vi "SENS_SEGM_STAT_ON_OFF.vi"(0 "VISA IN":refnum<visa-resource-name>, 1 "Segment":i32, 2 "Segment ON/OFF":bool, 5 "error in":errorcluster, 7 "Channel":i32) -> (14 "VISA Out":refnum<visa-resource-name>, 19 "error out":errorcluster)   [LabVIEW 2018, in "PNA-X.lvlib"]
doc: "SENSe<cnum>:SEGMent<snum>[:STATe] <ON | OFF> \n(Read-Write) Turns the specified sweep segment ON or OFF. At least ONE segment must be ON or \nSweep Mode is automatically set to Linear. \nParameters \n<cnum> Any existing channel number. If unspecified, value is set to 1 \n<snum> Segment number to be turned ON or OFF \n<ON | OFF> ON (or 1) - turns segment ON. \nOFF (or 0) - turns segment OFF. \nExamples SENS:SEGM ON \nsense2:segment2:state off \nQuery Syntax SENSe<cnum>:SEGMent<snum>[:STATe]? \nReturn Type Boolean (1 = ON, 0 = OFF) \nDefault OFF"
uses:
  PNA-X.lvlib
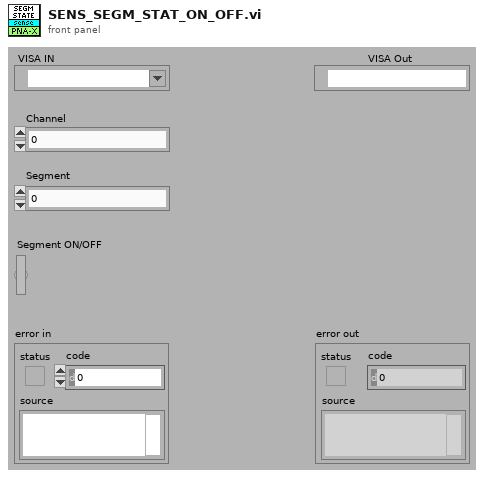
[diagram p1: front panel]
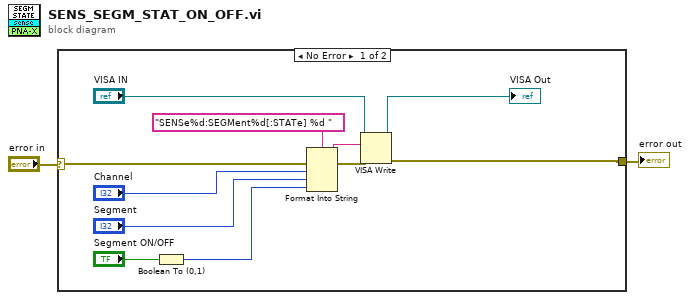
[diagram p0: block diagram]
diagram:
  n1 = case shown="No Error" "error in" {
    selector: "error in" -> [w13 w14]
    tunnel: [w8 w14] -> w1
    frame No Error {
      n2 = Boolean To (0,1)(Boolean="Segment ON/OFF") -> (0, 1=w3:i16)
      n3 = Format Into String(format string="SENSe%d:SEGMent%d[:STATe] %d " ("Cmdline"), error in=w13, "Channel", "Segment", w3) -> (resulting string=w11:string, error out=w12:errorcluster)  [unwired: 1 in]
      n4 = VISA Write(VISA resource name="VISA IN", write buffer=w11, error in (no error)=w12) -> (VISA resource name out=→"VISA Out":refnum<visa-resource-name>, error out=w8:errorcluster)  [unwired: 1 out]
    }
    frame Error {
    }
  }
  "error out" <- w1
